vi "SetSourceOffMode.vi"(7 "SMU":T1, 8 "Error In":errorcluster, 10 "Source Off Mode":T2, 11 "Keithley 2602 In":refnum<visa-resource-name>) -> (0 "Error Out":errorcluster, 3 "Keithley 2602 Out":refnum<visa-resource-name>)   [LabVIEW 2012, in "Keithley-2602.lvlib"]
uses:
  Keithley-2602.lvlib
  Controls/SourceOffMode.ctl
  Controls/SMU.ctl
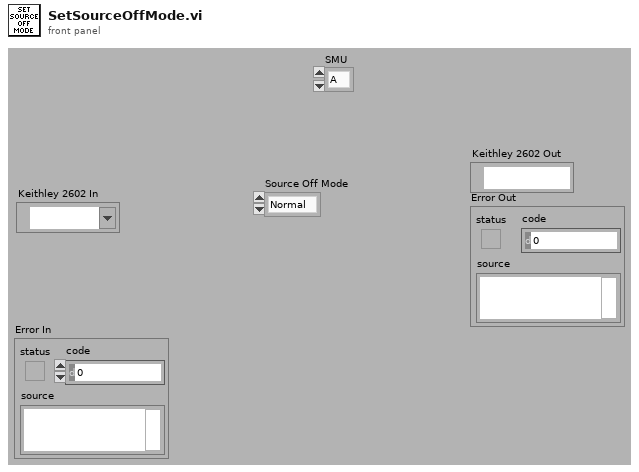
[diagram p1: front panel]
types:
  T1 = typedef "Keithley-2602.lvlib/SMU.ctl" = enum16{"A", "B"}
  T2 = typedef "Keithley-2602.lvlib/SourceOffMode.ctl" = enum16{"Normal", "Zero", "High Z"}
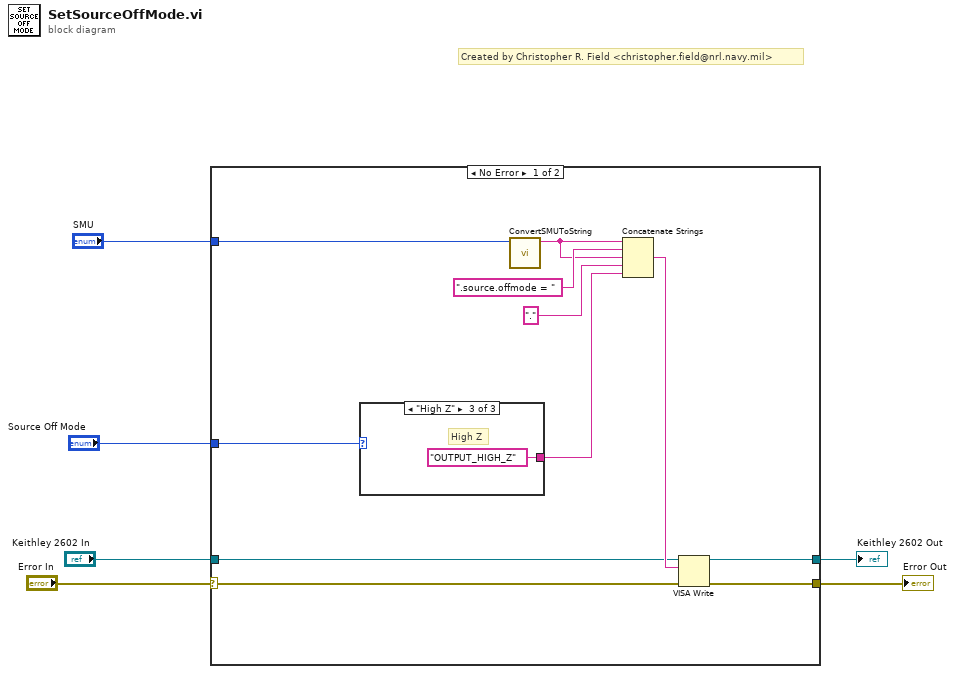
[diagram p0: block diagram]
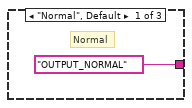
[diagram p2: hidden frame]
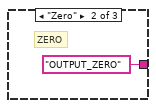
[diagram p3: hidden frame]
diagram:
  # "Created by Christopher R. Field <christopher.field@nrl.navy.mil>"
  n1 = case shown="No Error" "Error In" {
    selector: "Error In" -> [w7 w21]
    tunnel: "Keithley 2602 In" -> [w15 w22]
    tunnel: [w14 w22] -> w5
    tunnel: [w13 w21] -> w4
    tunnel: "SMU" -> [w9 _]
    tunnel: "Source Off Mode" -> [w8 _]
    frame No Error {
      n2 = case shown="\"High Z\"" w8 {
        tunnel: ["OUTPUT_NORMAL" "OUTPUT_ZERO" "OUTPUT_HIGH_Z"] -> w10
        frame "Normal", Default {
          # "Normal"
        }
        frame "Zero" {
          # "ZERO"
        }
        frame "High Z" {
          # "High Z"
        }
      }
      n3 = call "ConvertSMUToString.vi"("SMU"=w9) -> ("Channel"=w12:string)  [unwired: 10 in]
      n4 = Concatenate Strings(w12, ".source.offmode = ", w12, "." ("string"), w10) -> (w16:string)
      n5 = VISA Write(VISA resource name=w15, write buffer=w16, error in (no error)=w7) -> (VISA resource name out=w14:refnum<visa-resource-name>, error out=w13:errorcluster)  [unwired: 1 out]
    }
    frame Error {
    }
  }
  "Keithley 2602 Out" <- w5
  "Error Out" <- w4
